vi "SmartMotor UI Final.vi"() -> ()   [LabVIEW 2021]
panel:
  out "Console out":string
  out "intro":picture
  out "view":picture
  out "training 2":picture
  out "sent string":string
  out "training":u16[](array[numeric])
  out "Motor Value":i32
  in  "Quit":bool
  out "Training String":string
  out "Tab Control":enum32{"Welcome", "View", "Train"}(tab)
  in  "Ready":bool
  out "Motor Position View":u8(knob) scale=0.0..4.0
  in  "TRAIN":bool
  out "Sensor Intensity % View":dbl(slide) scale=0.0..100.0
  out "?":u32(colorbox)
  in  "Done":bool
  in  "?":bool
  in  "?":bool
  in  "?":bool
  in  "?":bool
  in  "Motor Position":u8(knob) scale=0.0..4.0
  out "Sensor Intensity %":dbl(slide) scale=0.0..100.0
  in  "Training Data":bool
  in  "Upload":bool
  out "Light Intensity 2":u32(colorbox)
  out "table":picture
  in  "Done 2":bool
  out "concatenated string":string
  out "read buffer":string
  out "Motor":string
  out "Sensor":string
  out "Type":string
  out "Name":string
  out "read terminal buffer - view":string
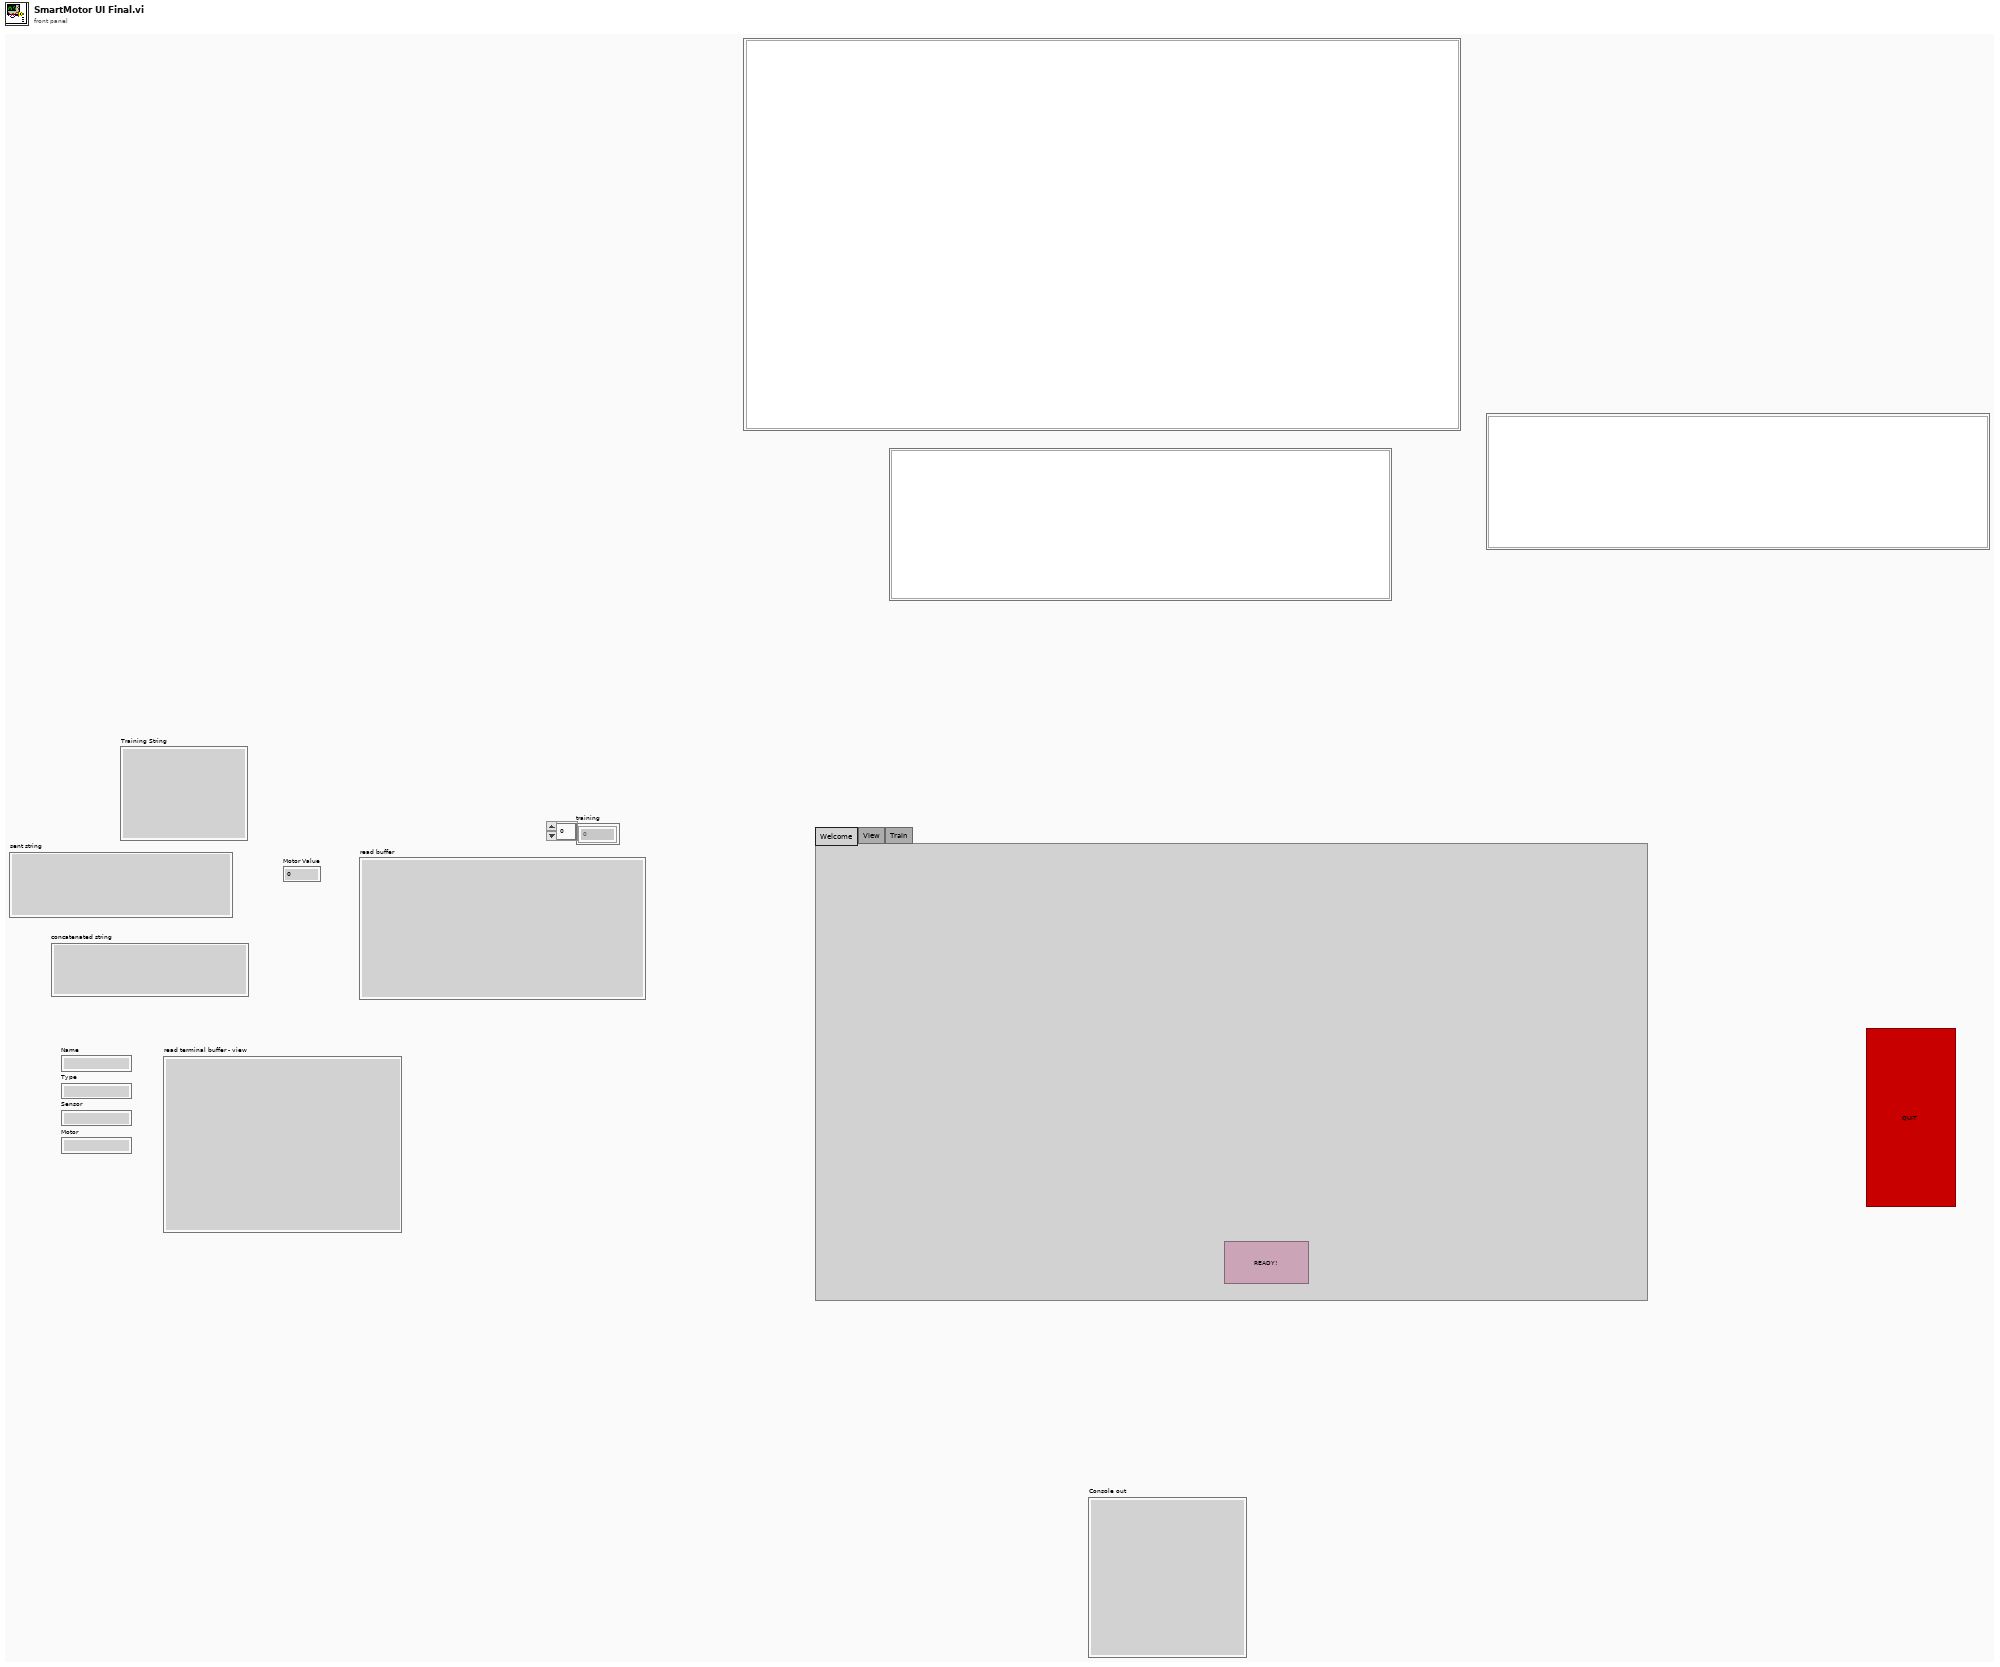
[diagram p1: front panel]
types:
  T1 = typedef "PythonCtrl.ctl" = cluster{"session":refnum<k35>, "PyPath":path, "Processor":enum16{"SPIKE", "Pi", "Pi_ssh"}}
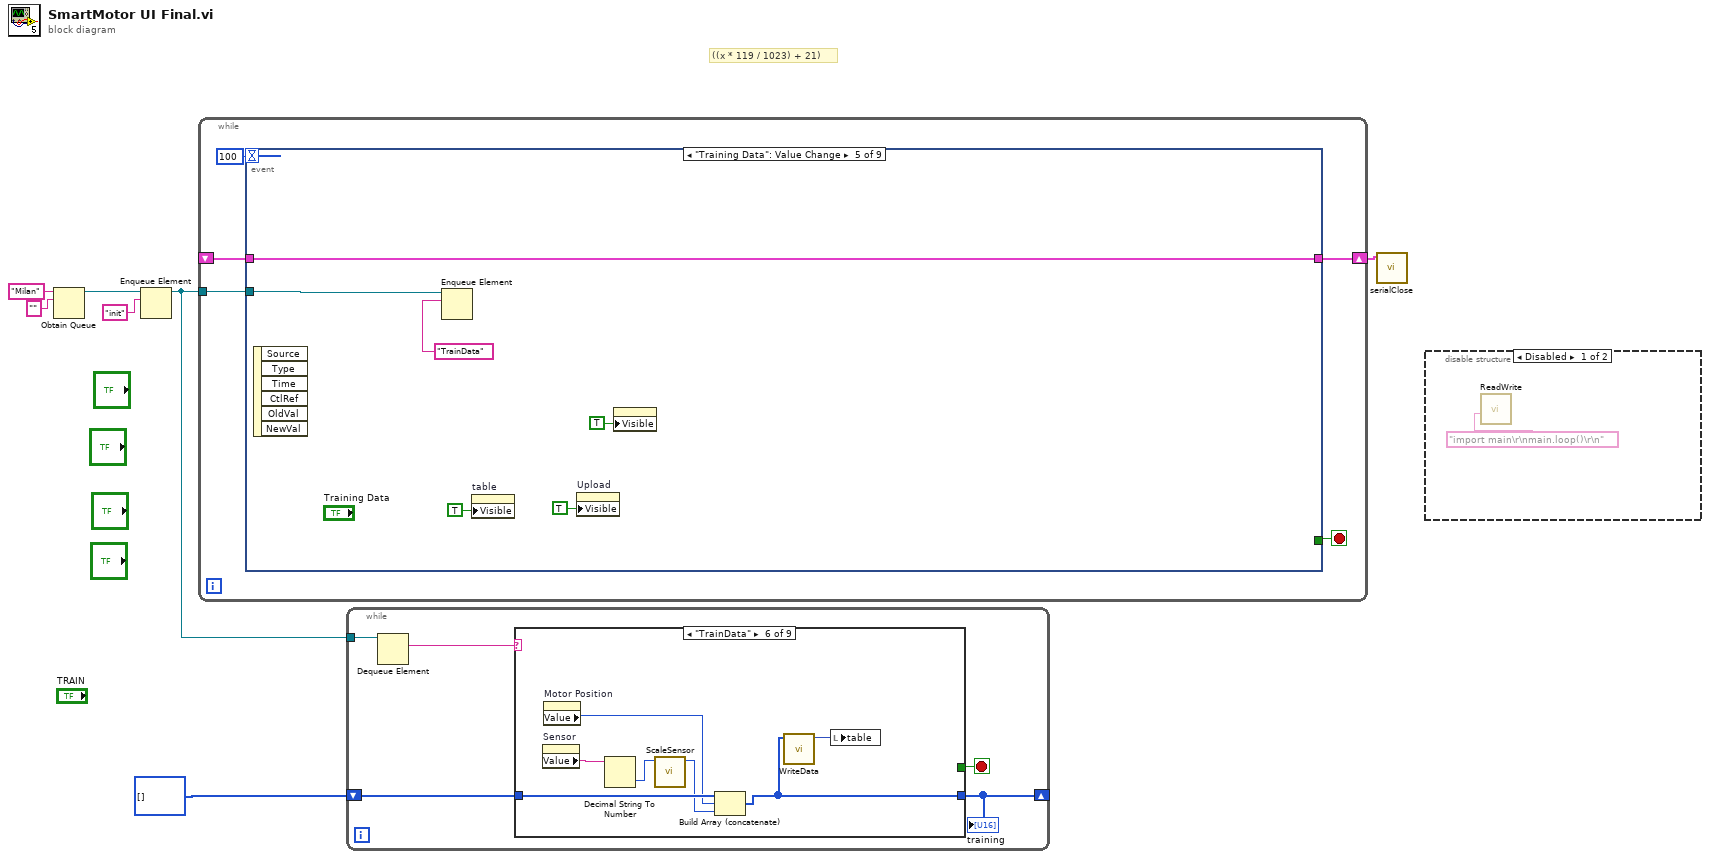
[diagram p0: block diagram]
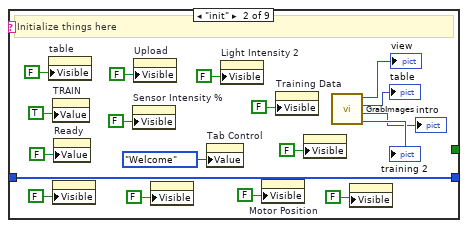
[diagram p4: hidden frame]
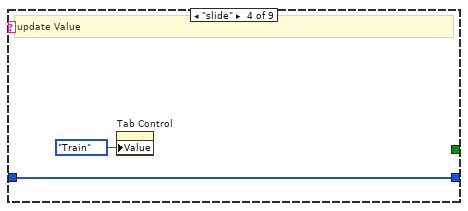
[diagram p6: hidden frame]
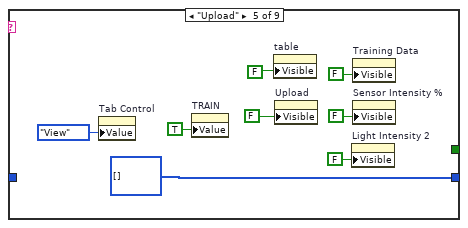
[diagram p7: hidden frame]
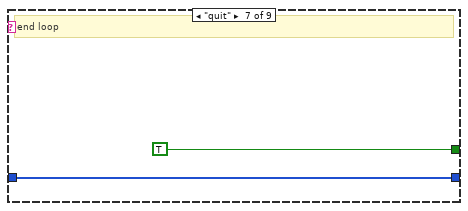
[diagram p8: hidden frame]
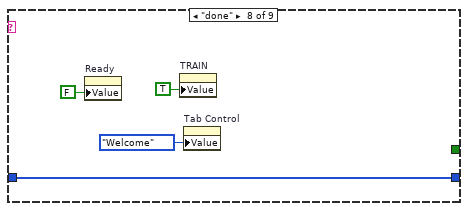
[diagram p9: hidden frame]
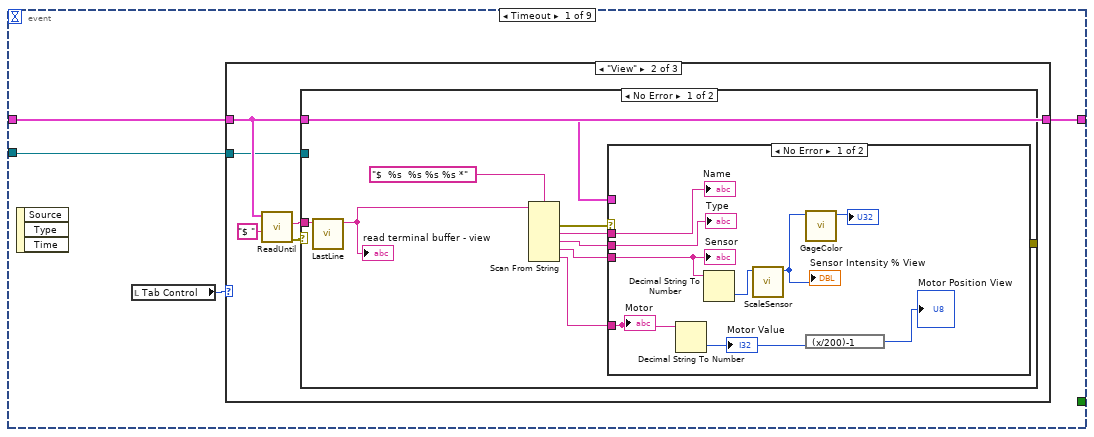
[diagram p11: hidden frame]
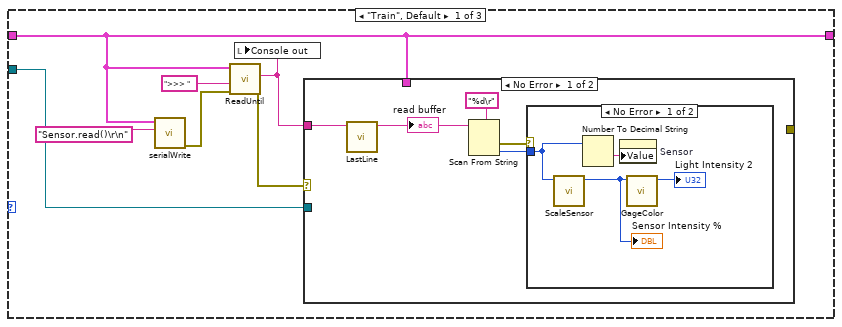
[diagram p12: hidden frame]
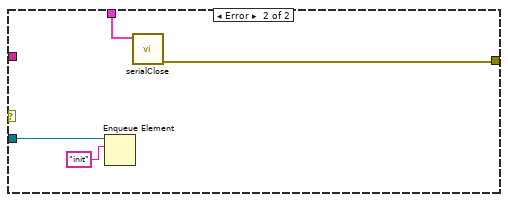
[diagram p14: hidden frame]
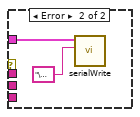
[diagram p15: hidden frame]
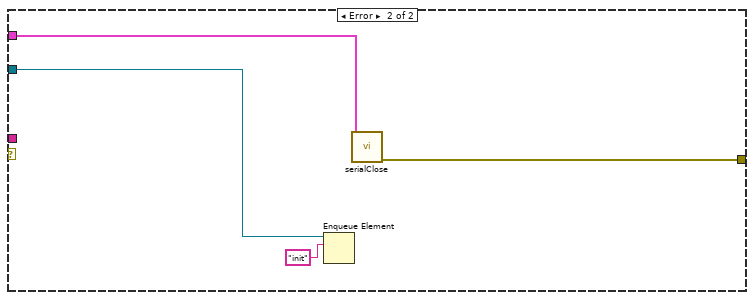
[diagram p16: hidden frame]
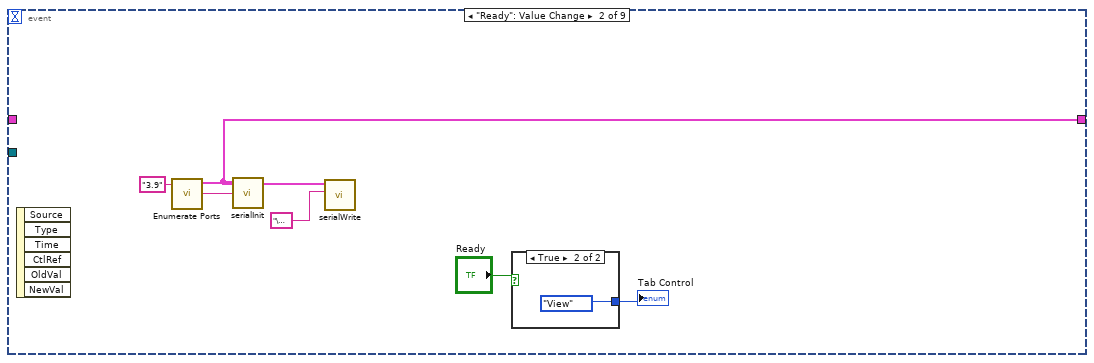
[diagram p18: hidden frame]
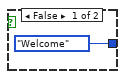
[diagram p19: hidden frame]
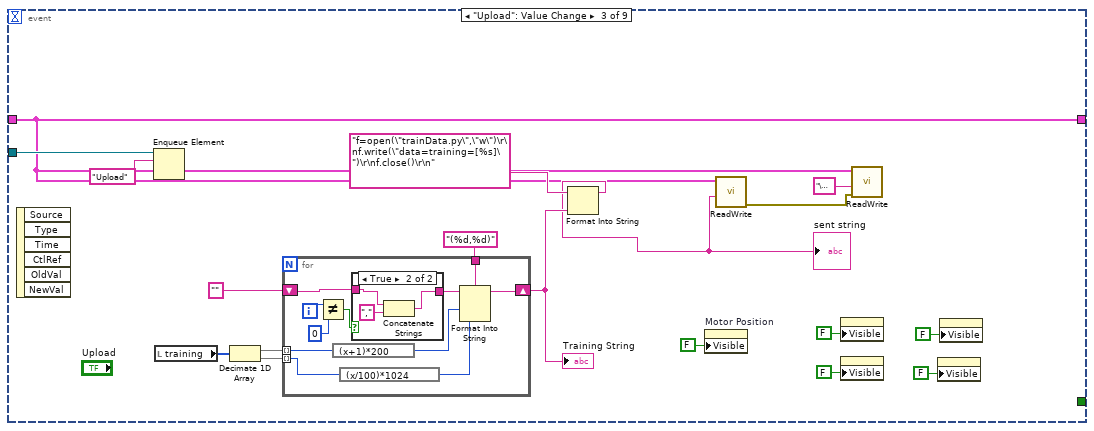
[diagram p20: hidden frame]
diagram:
  # "((x * 119 / 1023) + 21)"
  n1 = Obtain Queue(name (unnamed)="Milan", element data type="") -> (queue out=w7:refnum<queue>)  [unwired: 3 in, 2 out]
  n2 = Enqueue Element(queue=w7, element="init") -> (queue out=w3:refnum<queue>)  [unwired: 2 in, 2 out]
  n3 = while {
    tunnel: w3 -> [w12]
    shift-right: [w9] -> w2
    shift-left: _ -> [w10]
    stop <- w11 stop-if-true
    n4 = event shown="[4] \"Training Data\": Value Change" {
      selector: _ -> [_ _ _ _ _ _ _ _ _]
      dyn-events: _ -> [_ _ _ _ _ _ _ _ _]
      timeout: 100 -> [_ _ _ _ _ _ _ _ _]
      tunnel: w12 -> [w13 _ w92 _ w131 w143 w147 w151 w155]
      tunnel: [_ _ _ _ _ _ w146 TRUE ("Discard?") _] -> w11
      tunnel: w10 -> [w15 _ w80 w113 w130 w142 w145 w149 w153]
      tunnel: [w16 w67 w80 w111 w130 w142 w145 w149 w153] -> w9
      tunnel: [_ _ w80 _ _ _ _ _ _] -> _
      event Timeout {
        n5 = event-data() -> ()  [unwired: 1 in, 3 out]
        n6 = local read "Tab Control"() -> (w14:enum32{"Welcome", "View", "Train"})
        n7 = case shown="\"View\"" w14 {
          tunnel: w15 -> [w18 w41 w66]
          tunnel: [w18 w41 w66] -> w16
          tunnel: w13 -> [w17 w37 _]
          frame "Train", Default {
            n8 = call "serialWrite.vi"("text"="Sensor.read()\r\n" ("write buffer"), "Python"=w18) -> ("error out"=w21:errorcluster)  [unwired: 8 in, 1 out]
            n9 = call "ReadUntil.vi"("error in (no error)"=w21, "EOL"=">>> ", "Python"=w18) -> ("error out"=w19:errorcluster, "Console out"=w20:string)  [unwired: 6 in, 1 out]
            n10 = local write "Console out"(w20) -> ()
            n11 = case shown="No Error" w19 {
              tunnel: w20 -> [w24 _]
              tunnel: w18 -> [_ w35]
              tunnel: w17 -> [_ w34]
              tunnel: [_ w33] -> _
              frame No Error {
                n12 = call "LastLine.vi"("Reply"=w24) -> ("String"=w25:string)  [unwired: 10 in]
                "read buffer" <- w25
                n13 = Scan From String(format string="%d\r", input string=w25) -> (error out=w28:errorcluster, output 1=w27:i32)  [unwired: 3 in, 2 out]
                n14 = case shown="No Error" w28 {
                  tunnel: w27 -> [w30 _]
                  frame No Error {
                    n15 = call "ScaleSensor.vi"("value"=w30) -> ("scaled value"=w29:u16)  [unwired: 10 in]
                    "Sensor Intensity %" <- w29
                    n16 = Number To Decimal String(number=w30) -> (decimal integer string=w32:string)  [unwired: 1 in]
                    n17 = property on="Sensor" class="Str"("Value"=w32) -> ()  [unwired: 2 in, 2 out]
                    n18 = call "GageColor.vi"("value"=w29) -> ("Color Box"=→"Light Intensity 2":u32)  [unwired: 10 in]
                  }
                  frame Error {
                  }
                }
              }
              frame Error {
                n19 = Enqueue Element(queue=w34, element="init") -> ()  [unwired: 2 in, 3 out]
                n20 = call "serialClose.vi"("Python in"=w35) -> ("error out"=w33:errorcluster)  [unwired: 10 in]
              }
            }
          }
          frame "View" {
            n21 = call "ReadUntil.vi"("EOL"="$ ", "Python"=w41) -> ("error out"=w39:errorcluster, "Console out"=w40:string)  [unwired: 7 in, 1 out]
            n22 = case shown="No Error" w39 {
              tunnel: w40 -> [w44 _]
              tunnel: w41 -> [w42 w64]
              tunnel: w37 -> [_ w63]
              tunnel: [_ w62] -> _
              frame No Error {
                n23 = call "LastLine.vi"("Reply"=w44) -> ("String"=w43:string)  [unwired: 10 in]
                "read terminal buffer - view" <- w43
                n24 = Scan From String(format string="$  %s  %s %s %s *", input string=w43) -> (error out=w50:errorcluster, output 1=w46:string, output 2=w47:string, output 3=w48:string, output 4=w49:string)  [unwired: 6 in, 2 out]
                n25 = case shown="No Error" w50 {
                  tunnel: w46 -> [w59 _]
                  tunnel: w47 -> [w58 _]
                  tunnel: w48 -> [w57 _]
                  tunnel: w49 -> [w54 _]
                  tunnel: w42 -> [_ w61]
                  frame No Error {
                    n26 = Decimal String To Number(string=w54) -> (number=w52:i32)  [unwired: 2 in, 1 out]
                    "Motor Value" <- w52
                    n27 = Decimal String To Number(string=w57) -> (number=w56:i32)  [unwired: 2 in, 1 out]
                    n28 = call "ScaleSensor.vi"("value"=w56) -> ("scaled value"=w53:u16)  [unwired: 10 in]
                    "Sensor Intensity % View" <- w53
                    n29 = call "GageColor.vi"("value"=w53) -> ("Color Box"=→"?":u32)  [unwired: 10 in]
                    n30 = expression code="(x/200)-1"(w52) -> (→"Motor Position View":i32)
                    "Name" <- w59
                    "Type" <- w58
                    "Sensor" <- w57
                    "Motor" <- w54
                  }
                  frame Error {
                    n31 = call "serialWrite.vi"("text"="\u0003", "Python"=w61) -> ()  [unwired: 8 in, 2 out]
                  }
                }
              }
              frame Error {
                n32 = Enqueue Element(queue=w63, element="init") -> ()  [unwired: 2 in, 3 out]
                n33 = call "serialClose.vi"("Python in"=w64) -> ("error out"=w62:errorcluster)  [unwired: 10 in]
              }
            }
          }
          frame "Welcome" {
          }
        }
      }
      event "Ready": Value Change {
        n34 = event-data() -> ()  [unwired: 1 in, 6 out]
        n35 = call "Enumerate Ports.vi"("Python version"="3.9") -> ("guess"=w70:string, "Python"=w67:T1)  [unwired: 6 in, 3 out]
        n36 = call "serialInit.vi"("Port"=w70, "Python"=w67) -> ()  [unwired: 8 in, 2 out]
        n37 = call "serialWrite.vi"("text"="\u0004" ("write buffer"), "Python"=w67) -> ()  [unwired: 8 in, 2 out]
        n38 = case shown="True" "Ready" {
          tunnel: [enum32{"Welcome", "View", "Train"}."Welcome" ("Tab Control") enum32{"Welcome", "View", "Train"}."View" ("Tab Control")] -> w71
          frame False {
          }
          frame True {
          }
        }
        "Tab Control" <- w71
      }
      event "Upload": Value Change {
        n39 = event-data() -> ()  [unwired: 1 in, 6 out]
        n40 = Enqueue Element(queue=w92, element="Upload") -> ()  [unwired: 2 in, 3 out]
        n41 = local read "training"() -> (w90:u16[])
        n42 = Decimate 1D Array(w90) -> (w88:u16[], w87:u16[])
        n43 = for {
          tunnel: "(%d,%d)" ("format string") -> [w103]
          tunnel: w88 -> [w96] mode=indexing
          tunnel: w87 -> [w94] mode=indexing
          shift-right: [w102] -> w85
          shift-left: "" -> [w101]
          i -> [w98]
          n44 = Not Equal?(x=w98, y=0) -> (x != y?=w99:bool)
          n45 = expression code="(x+1)*200"(w96) -> (w95:u16)
          n46 = expression code="(x/100)*1024"(w94) -> (w93:u16)
          n47 = case shown="True" w99 {
            tunnel: w101 -> [w104 w106]
            tunnel: [w104 w105] -> w100
            frame False {
            }
            frame True {
              n48 = Concatenate Strings(w106, "," ("string")) -> (w105:string)
            }
          }
          n49 = Format Into String(format string=w103, initial string=w100, w95, w93) -> (resulting string=w102:string)  [unwired: 1 in, 1 out]
        }
        "Training String" <- w85
        n50 = Format Into String(format string="f=open(\"trainData.py\",\"w\")\r\nf.write(\"data=training=[%s]\")\r\nf.close()\r\n" ("string"), w85) -> (resulting string=w83:string)  [unwired: 2 in, 1 out]
        "sent string" <- w83
        n51 = property on="Motor Position" class="Knob (strict)"("Visible"=FALSE) -> ()  [unwired: 2 in, 2 out]
        n52 = call "ReadWrite.vi"("Code"=w83, "Python"=w80) -> ("error out"=w81:errorcluster)  [unwired: 8 in, 1 out]
        n53 = property class="Bool"("Visible"=FALSE) -> ()  [unwired: 2 in, 2 out]
        n54 = property class="Bool"("Visible"=FALSE) -> ()  [unwired: 2 in, 2 out]
        n55 = call "ReadWrite.vi"("error in (no error)"=w81, "Code"="\u0004" ("text"), "Python"=w80) -> ()  [unwired: 7 in, 2 out]
        n56 = property class="Bool"("Visible"=FALSE) -> ()  [unwired: 2 in, 2 out]
        n57 = property class="Bool"("Visible"=FALSE) -> ()  [unwired: 2 in, 2 out]
      }
      event "TRAIN": Value Change {
        # "Hit btn on Front Panel"
        n58 = event-data() -> ()  [unwired: 1 in, 1 out]
        n59 = property on="Tab Control" class="TabCtl (strict)"("Value"=enum32{"Welcome", "View", "Train"}."Train" ("Tab Control")) -> ()  [unwired: 2 in, 2 out]
        n60 = for {
          N: 5 -> [_]
          shift-right: [w116] -> w111
          shift-left: w113 -> [w118]
          tunnel: [w115] -> w109
          i -> [w115]
          n61 = while {
            tunnel: w118 -> [w121]
            tunnel: [w121] -> w116
            shift-right: [w120] -> _
            shift-left: "" ("Console out") -> [w119]
            stop <- w123 continue-if-true
            # "Make sure that the CtrlC catches"
            n62 = call "serialWrite.vi"("text"="\u0003" ("write buffer"), "Python"=w121) -> ("error out"=w124:errorcluster)  [unwired: 8 in, 1 out]
            n63 = Wait (ms)(milliseconds to wait=u32 500) -> ()  [unwired: 1 out]
            n64 = call "ReadUntil.vi"("error in (no error)"=w124, "EOL"=">>> ", "Console in"=w119, "Python"=w121) -> ("timed out?"=w123:bool, "Console out"=w120:string)  [unwired: 5 in, 1 out]
            "Console out" <- w120
          }
        }
        n65 = Equal?(x=w109, y=4.0) -> (x = y?=w108:bool)
        n66 = property class="Bool"("Visible"=w108) -> ()  [unwired: 2 in, 2 out]
        n67 = property on="Motor Position" class="Knob (strict)"("Visible"=w108) -> ()  [unwired: 2 in, 2 out]
      }
      event "Training Data": Value Change {
        n68 = event-data() -> ()  [unwired: 1 in, 6 out]
        n69 = Enqueue Element(queue=w131, element="TrainData") -> ()  [unwired: 2 in, 3 out]
        n70 = property on="table" class="Pict"("Visible"=TRUE) -> ()  [unwired: 2 in, 2 out]
        n71 = property on="Upload" class="Bool (strict)"("Visible"=TRUE) -> ()  [unwired: 2 in, 2 out]
        n72 = property class="Bool"("Visible"=TRUE) -> ()  [unwired: 2 in, 2 out]
      }
      event "Motor Position": Value Change {
        # "Slide slid on Front Panel"
        n73 = event-data() -> ()  [unwired: 1 in, 6 out]
        n74 = Enqueue Element(queue=w143, element="slide") -> ()  [unwired: 2 in, 3 out]
        n75 = property class="Bool"("Visible"=TRUE) -> ()  [unwired: 2 in, 2 out]
        n76 = property on="Training Data" class="Bool"("Visible"=TRUE) -> ()  [unwired: 2 in, 2 out]
        n77 = expression code="(x+1)*30"("Motor Position") -> (w138:u8)
        n78 = Format Into String(format string="pwm2.duty(%d)\r\n", w138) -> (resulting string=w140:string)  [unwired: 2 in, 1 out]
        "concatenated string" <- w140
        n79 = property on="Sensor Intensity %" class="Slide (strict)"("Visible"=TRUE) -> ()  [unwired: 2 in, 2 out]
        n80 = property class="Bool"("Visible"=TRUE) -> ()  [unwired: 2 in, 2 out]
        n81 = call "serialWrite.vi"("text"=w140, "Python"=w142) -> ()  [unwired: 8 in, 2 out]
        n82 = property on="Light Intensity 2" class="ColBox"("Visible"=TRUE) -> ()  [unwired: 2 in, 2 out]
      }
      event Panel Close? {
        w146 = TRUE ("Discard?")
        # "Closed the Window"
        n83 = event-data() -> ()  [unwired: 1 in, 2 out]
        n84 = Enqueue Element(queue=w147, element="done") -> ()  [unwired: 2 in, 3 out]
        n85 = event-data("Discard?"=w146) -> ()  [unwired: 1 in, 1 out]
      }
      event "Quit": Value Change {
        # "hit Done btn"
        n86 = event-data() -> ()  [unwired: 1 in, 2 out]
        n87 = Enqueue Element(queue=w151, element="quit") -> ()  [unwired: 2 in, 3 out]
      }
      event "Done", "Done 2": Value Change {
        n88 = event-data() -> ()  [unwired: 1 in, 6 out]
        n89 = Enqueue Element(queue=w155, element="done") -> ()  [unwired: 2 in, 3 out]
        n90 = call "ReadWrite.vi"("Code"="\u0004" ("text"), "Python"=w153) -> ()  [unwired: 8 in, 2 out]
      }
    }
  }
  n91 = while {
    tunnel: w3 -> [w161]
    shift-right: [w157] -> _
    shift-left: u16[] [] ("initialized array") -> [w158]
    stop <- w159 stop-if-true
    n92 = Dequeue Element(queue=w161) -> (element=w160:string)  [unwired: 2 in, 3 out]
    n93 = case shown="\"TrainData\"" w160 {
      tunnel: [_ _ _ _ _ _ TRUE ("Discard?") _ _] -> w159
      tunnel: w158 -> [w162 w180 w181 w183 _ w198 w199 w203 w205]
      tunnel: [w162 w180 w181 w183 u16[] [] ("initialized array") w194 w199 w203 w205] -> w157
      frame Default {
      }
      frame "init" {
        # "Initialize things here"
        n94 = property on="table" class="Pict"("Visible"=FALSE) -> ()  [unwired: 2 in, 2 out]
        n95 = property on="TRAIN" class="Bool (strict)"("Value"=TRUE ("Train")) -> ()  [unwired: 2 in, 2 out]
        n96 = property class="Bool"("Visible"=FALSE) -> ()  [unwired: 2 in, 2 out]
        n97 = property on="Ready" class="Bool (strict)"("Value"=FALSE ("Ready")) -> ()  [unwired: 2 in, 2 out]
        n98 = property on="Sensor Intensity %" class="Slide (strict)"("Visible"=FALSE) -> ()  [unwired: 2 in, 2 out]
        n99 = property on="Upload" class="Bool (strict)"("Visible"=FALSE) -> ()  [unwired: 2 in, 2 out]
        n100 = property class="Bool"("Visible"=FALSE) -> ()  [unwired: 2 in, 2 out]
        n101 = property on="Tab Control" class="TabCtl (strict)"("Value"=enum32{"Welcome", "View", "Train"}."Welcome" ("Tab Control")) -> ()  [unwired: 2 in, 2 out]
        n102 = property on="Light Intensity 2" class="ColBox"("Visible"=FALSE) -> ()  [unwired: 2 in, 2 out]
        n103 = property on="Motor Position" class="Knob (strict)"("Visible"=FALSE) -> ()  [unwired: 2 in, 2 out]
        n104 = property on="Training Data" class="Bool"("Visible"=FALSE) -> ()  [unwired: 2 in, 2 out]
        n105 = property class="Bool"("Visible"=FALSE) -> ()  [unwired: 2 in, 2 out]
        n106 = call "GrabImages.vi"() -> ("Training Instructions"=→"training 2":picture, "Intro"=→"intro":picture, "Table"=→"table":picture, "View Instructions"=→"view":picture)  [unwired: 8 in]
        n107 = property class="Bool"("Visible"=FALSE) -> ()  [unwired: 2 in, 2 out]
      }
      frame "Train" {
        # "reset LED"
      }
      frame "slide" {
        # "update Value"
        n108 = property on="Tab Control" class="TabCtl (strict)"("Value"=enum32{"Welcome", "View", "Train"}."Train" ("Tab Control")) -> ()  [unwired: 2 in, 2 out]
      }
      frame "Upload" {
        n109 = property on="Tab Control" class="TabCtl (strict)"("Value"=enum32{"Welcome", "View", "Train"}."View" ("Tab Control")) -> ()  [unwired: 2 in, 2 out]
        n110 = property on="TRAIN" class="Bool (strict)"("Value"=TRUE ("TRAIN")) -> ()  [unwired: 2 in, 2 out]
        n111 = property on="table" class="Pict"("Visible"=FALSE) -> ()  [unwired: 2 in, 2 out]
        n112 = property on="Upload" class="Bool (strict)"("Visible"=FALSE) -> ()  [unwired: 2 in, 2 out]
        n113 = property on="Light Intensity 2" class="ColBox"("Visible"=FALSE) -> ()  [unwired: 2 in, 2 out]
        n114 = property on="Training Data" class="Bool"("Visible"=FALSE) -> ()  [unwired: 2 in, 2 out]
        n115 = property on="Sensor Intensity %" class="Slide (strict)"("Visible"=FALSE) -> ()  [unwired: 2 in, 2 out]
      }
      frame "TrainData" {
        n116 = property on="Sensor" class="Str"() -> ("Value"=w197:string)  [unwired: 2 in, 2 out]
        n117 = property on="Motor Position" class="Knob (strict)"() -> ("Value"=w192:u8)  [unwired: 2 in, 2 out]
        n118 = Decimal String To Number(string=w197) -> (number=w196:i32)  [unwired: 2 in, 1 out]
        n119 = call "ScaleSensor.vi"("value"=w196) -> ("scaled value"=w195:u16)  [unwired: 10 in]
        n120 = Build Array (concatenate)(w198, w192, w195) -> (w194:u16[])
        n121 = call "WriteData.vi"("Array"=w194) -> ("Table"=w193:picture)  [unwired: 10 in]
        n122 = local write "table"(w193) -> ()
      }
      frame "quit" {
        # "end loop"
      }
      frame "done" {
        n123 = property on="Ready" class="Bool (strict)"("Value"=FALSE ("Ready")) -> ()  [unwired: 2 in, 2 out]
        n124 = property on="TRAIN" class="Bool (strict)"("Value"=TRUE ("TRAIN")) -> ()  [unwired: 2 in, 2 out]
        n125 = property on="Tab Control" class="TabCtl (strict)"("Value"=enum32{"Welcome", "View", "Train"}."Welcome" ("Tab Control")) -> ()  [unwired: 2 in, 2 out]
      }
      frame "" {
      }
    }
    "training" <- w157
  }
  n126 = call "serialClose.vi"("Python in"=w2) -> ()  [unwired: 10 in, 1 out]
  n127 = disable-structure shown="Disabled" {
    frame Disabled {
      n128 = call "ReadWrite.vi"("Code"="import main\r\nmain.loop()\r\n" ("text")) -> ()  [unwired: 9 in, 2 out]
    }
    frame Enabled {
    }
  }
